vi "debug.vi"   [LabVIEW 2015]
uses:
  <vilib>/Utility/file.llb/Write Delimited Spreadsheet (DBL).vi
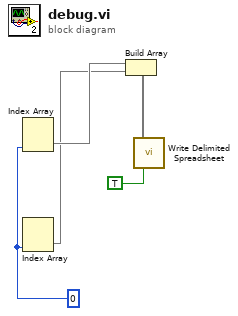
[diagram p0: block diagram]
diagram:
  w1 = 0
  n1 = Index Array(index (col)=w1) -> (array=w7:dbl[][], element=w4)  [unwired: 1 in]
  n2 = Index Array(index (col)=w1) -> (array=w6:dbl[][], element=w3)  [unwired: 1 in]
  n3 = Build Array(w4, w3) -> (w2:void[])
  n4 = call-poly <vilib>:"Write Delimited Spreadsheet.vi"("2D data"=w2, "transpose? (F)"=TRUE) -> ()  [unwired: 12 in, 2 out]
